vi "pack.vi"(8 "error in (no error)":errorcluster, 11 "K2602FileReader in":refnum<class "K2602FileReader.lvclass">) -> (0 "error out":errorcluster, 3 "K2602FileReader out":refnum<class "K2602FileReader.lvclass">)   [LabVIEW 2011, in "Tools.lvlib" / "Filing.lvlib" / "K2602FileReader.lvclass"]
uses:
  K2602FileReader.lvclass
  K2602FileReader.lvclass/K2602FileReader.ctl
  FileReader.lvclass
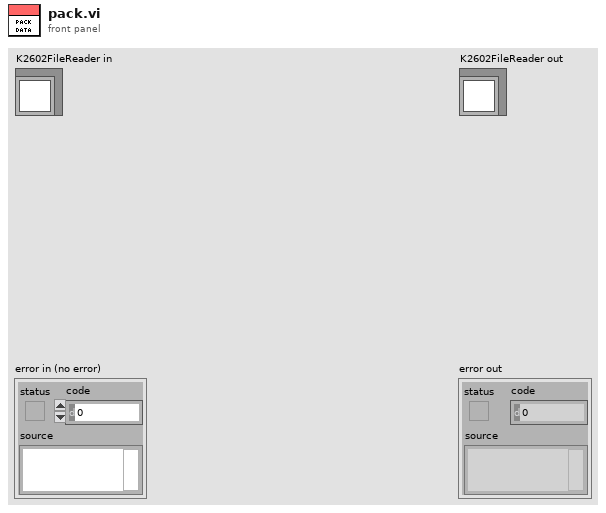
[diagram p1: front panel]
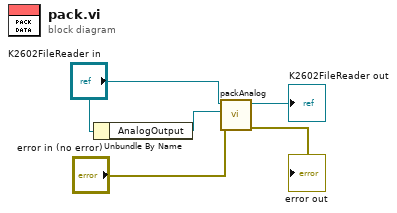
[diagram p0: block diagram]
diagram:
  n1 = Unbundle By Name("K2602FileReader in") -> ("AnalogOutput"=w4:refnum<class "AnalogOutput.lvclass">)
  n2 = call "packAnalog.vi"("error in (no error)"="error in (no error)", "AnalogOutput"=w4, "FileReader in"="K2602FileReader in") -> ("error out"=→"error out":errorcluster, "FileReader out"=→"K2602FileReader out":refnum<class "K2602FileReader.lvclass">)  [unwired: 7 in]
